vi "Math Algos 2.vi"(9 "Measurements 2":T1, 11 "W (from Top View Algo)":dbl[](array[numeric]) format="%#_13g") -> (3 "H corrected":dbl[](array[numeric]))   [LabVIEW 2019, in "Algorithm.lvclass"]
uses:
  FrameworkOverrides/Algorithm.lvclass
  Controls/Measurements JSON Read.ctl
panel:
  out "NumericAray":i32[][](array[numeric])
  out "MeasurementIndices":i32[][](array[numeric])
  out "Array":string[](array[string])
  out "Alpha":dbl[](array[numeric])
  out "Thickness":dbl[](array[numeric])
  out "CurlGap":dbl[](array[numeric])
  out "Radius":dbl[](array[numeric])
  out "CamID":i32[](array[numeric])=[0, 0, 0, 1, 2, 1, 2, 1, 2, 1, 2, 0, 1, 2, 1, 2]
  out "Htrig":dbl[](array[numeric])
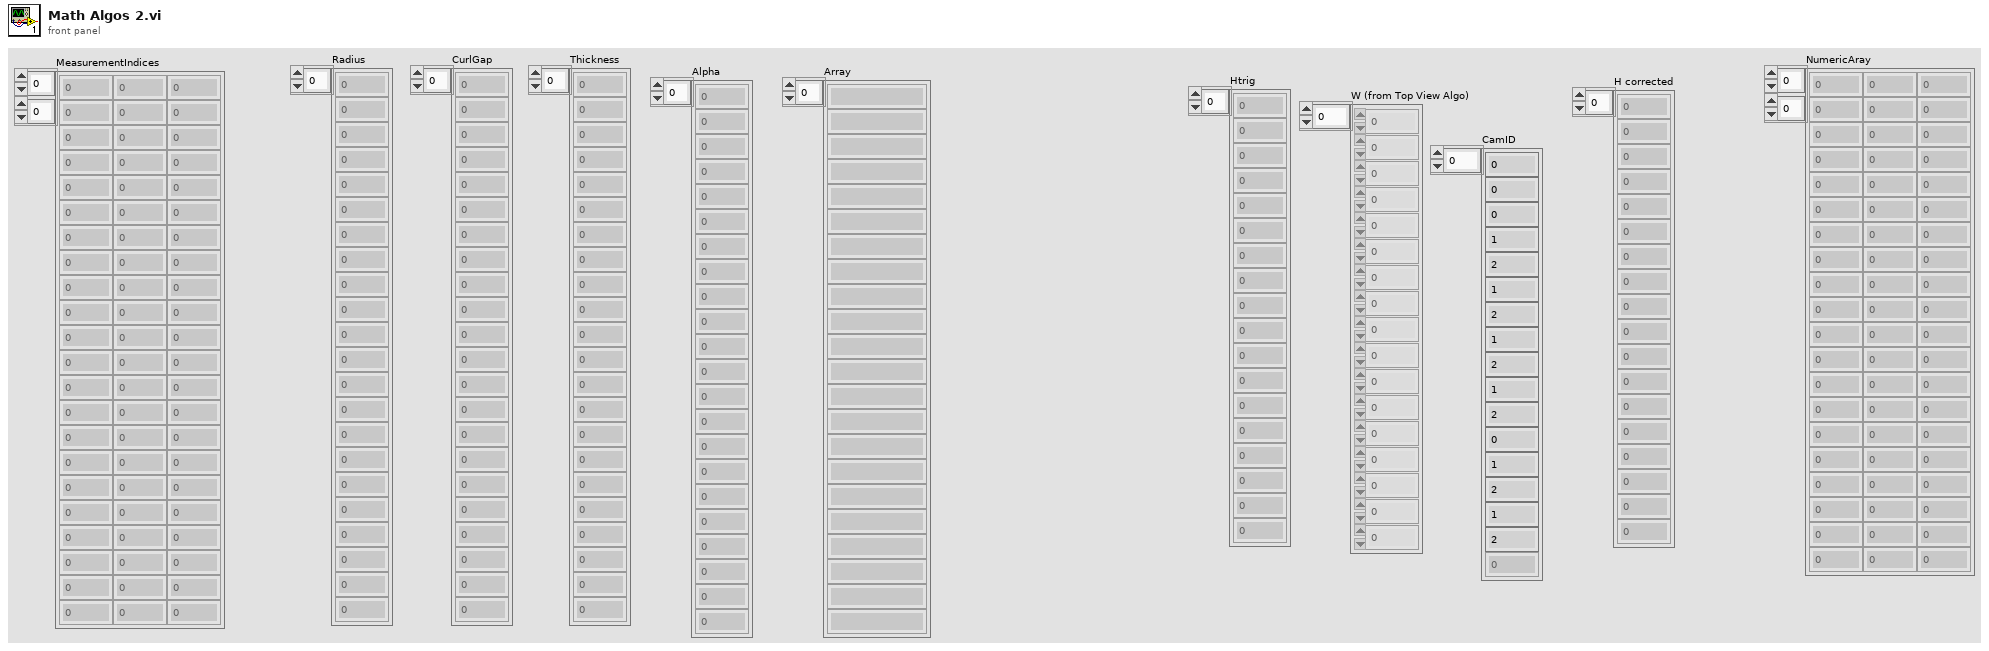
[diagram p1: front panel]
types:
  T1 = typedef "Algorithm.lvclass/Measurements JSON Read.ctl" = cluster{"RackID":i32, "ImageID":i32, "CameraID":i32, "MeasurementId":i32, "Name":string, "AlgoName":string, "Type":string, "MeasurementEnable":bool, "AlgorithmSequence":cluster{"RefernceEdge":cluster{"Enable":bool, "Method":string, "RefROI":cluster{"Left":i32, "Top":i32, "Right":i32, "Bottom":i32, "Rotation":dbl}, "EdgeOptions":cluster{"EdgePoarity":i32, "KernelSize":i32, "Width":i32, "MinimumEdgeStrength":i32, "InterpolationType":i32, "DataProcessingMethod":i32}, "LineOptions":cluster{"NumberofLines":i32, "Type":i32, "MinScore":i32, "MaxScore":i32, "Orientation":i32, "AngleRange":i32, "AngleTolerance":i32, "StepSize":i32, "MinSNR":i32, "MinPoints":i32, "HoughIterations":i32}, "SearchDirection":i32}, "Measurement":cluster{"ROI1":cluster{"Enable":bool, "ROI":cluster{"Left":i32, "Top":i32, "Right":i32, "Bottom":i32, "Rotation":dbl}, "EdgeOptions":cluster{"EdgePoarity":i32, "KernelSize":i32, "Width":i32, "MinimumEdgeStrength":i32, "InterpolationType":i32, "DataProcessingMethod":i32}, "LineOptions":cluster{"NumberofLines":i32, "Type":i32, "MinScore":i32, "MaxScore":i32, "Orientation":i32, "AngleRange":i32, "AngleTolerance":i32, "StepSize":i32, "MinSNR":i32, "MinPoints":i32, "HoughIterations":i32}, "Process":i32, "StepSize":i32, "SearchDirection":i32, "CircleEdgeOptions":cluster{"SearchDirection":i32, "EdgeOptions":cluster{"EdgePoarity":i32, "KernelSize":i32, "Width":i32, "MinimumEdgeStrength":i32, "InterpolationType":i32, "DataProcessingMethod":i32}}, "CircleFitOptions":cluster{"Process":i32, "StepSize":i32, "MAxPixelRadius":dbl}, "CircleSearchDirection":i32, "CurveParameters":cluster{"ExtractionMode":i32, "EdgeThreshold":i32, "EdgeFilterSize":i32, "MinLength":i32, "RowSearchStepSize":i32, "ColSearchStepSize":i32, "MaxEndpointGap":i32, "Closed":bool, "Subpixel":bool}, "MinimumMatchScore":i32, "CircleDescriptor":cluster{"MinRadius":i32, "MaxRadius":i32}, "EllipseDescriptor":cluster{"MinMajorRadius":i32, "MaxMajorRadius":i32, "MinMinorRadius":i32, "MaxMinorRadius":i32}}, "ROI2":cluster{"Enable":bool, "ROI":cluster{"Left":i32, "Top":i32, "Right":i32, "Bottom":i32, "Rotation":dbl}, "EdgeOptions":cluster{"EdgePoarity":i32, "KernelSize":i32, "Width":i32, "MinimumEdgeStrength":i32, "InterpolationType":i32, "DataProcessingMethod":i32}, "LineOptions":cluster{"NumberofLines":i32, "Type":i32, "MinScore":i32, "MaxScore":i32, "Orientation":i32, "AngleRange":i32, "AngleTolerance":i32, "StepSize":i32, "MinSNR":i32, "MinPoints":i32, "HoughIterations":i32}, "Process":i32, "StepSize":i32, "SearchDirection":i32, "CircleEdgeOptions":cluster{"SearchDirection":i32, "EdgeOptions":cluster{"EdgePoarity":i32, "KernelSize":i32, "Width":i32, "MinimumEdgeStrength":i32, "InterpolationType":i32, "DataProcessingMethod":i32}}, "CircleFitOptions":cluster{"Process":i32, "StepSize":i32, "MAxPixelRadius":dbl}, "CircleSearchDirection":i32, "CurveParameters":cluster{"ExtractionMode":i32, "EdgeThreshold":i32, "EdgeFilterSize":i32, "MinLength":i32, "RowSearchStepSize":i32, "ColSearchStepSize":i32, "MaxEndpointGap":i32, "Closed":bool, "Subpixel":bool}, "MinimumMatchScore":i32, "CircleDescriptor":cluster{"MinRadius":i32, "MaxRadius":i32}, "EllipseDescriptor":cluster{"MinMajorRadius":i32, "MaxMajorRadius":i32, "MinMinorRadius":i32, "MaxMinorRadius":i32}}}}, "MathExpression":cluster{"Algorithm":string, "MathExpression":string, "ResultVariable":string}, "MathCorrectionParameters":cluster{"Radius":dbl, "CurlGap":dbl, "Thickness":dbl, "MeasurementIndices":i32[], "MathAlgoName":string, "MathAlgoFormula":string, "CorrectionForAngle":i32[], "NumericAray":i32[], "StringArray":string[]}, "ResultVariableCluster":cluster{"RVName":string, "RVSequence":string, "RVIndex":i32, "RVID":i32, "RVValue":dbl}, "CalibrationCoefficients":cluster{"A1":dbl, "A2":dbl, "A3":dbl}, "UserCalibCoefficients":cluster{"UserCorrectionLinearityCoeff":dbl, "UserCorrectionBiasCoeff":dbl}, "SpecValues":cluster{"LCL":dbl, "UCL":dbl, "LSL":dbl, "USL":dbl, "NominalValue":dbl}, "OverlayOptions":cluster{"OverlayEnable":bool, "OverlayText":string, "OverlayCoords":i32[], "OverlayAngle":i32, "OverlayTextSize":i32, "OverlayTextColor":string, "OverlayROI":bool, "OverlayRakeLine":bool, "OverlayPoints":bool}, "DatalogEnable":bool, "DisplayIcon":string}[]
  T2 = cluster{"Radius":dbl, "CurlGap":dbl, "Thickness":dbl, "MeasurementIndices":i32[], "MathAlgoName":string, "MathAlgoFormula":string, "CorrectionForAngle":i32[], "NumericAray":i32[], "StringArray":string[]}
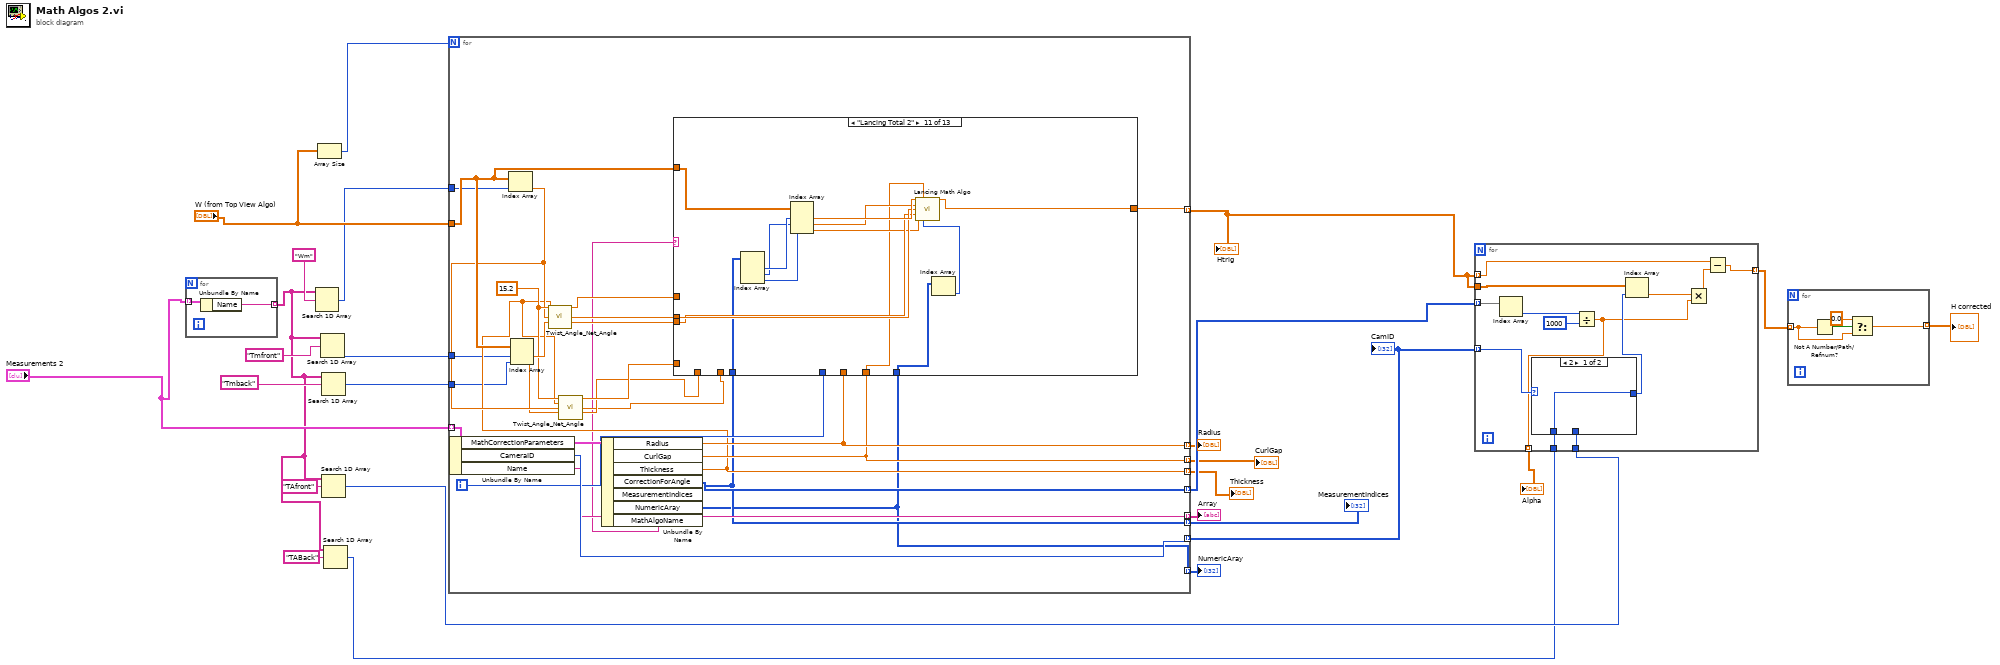
[diagram p0: block diagram]
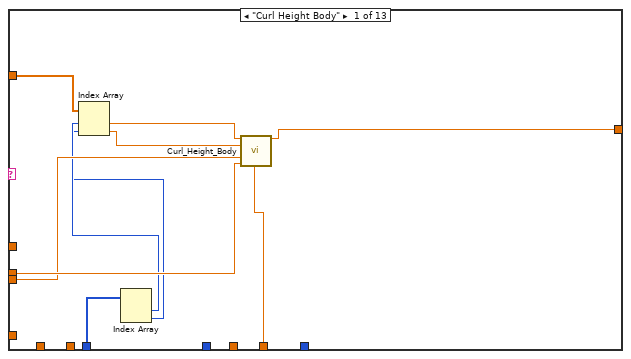
[diagram p3: hidden frame]
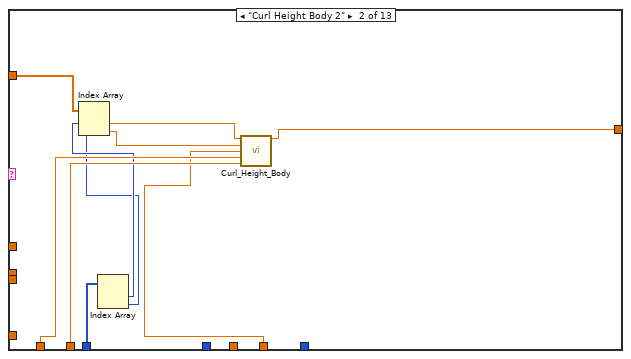
[diagram p4: hidden frame]
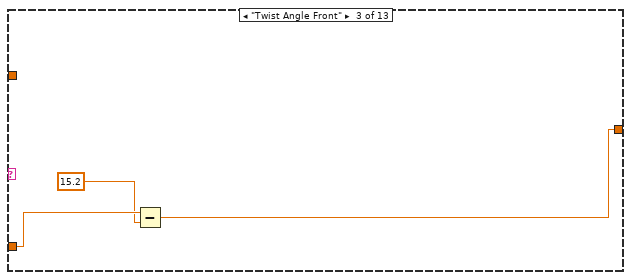
[diagram p5: hidden frame]
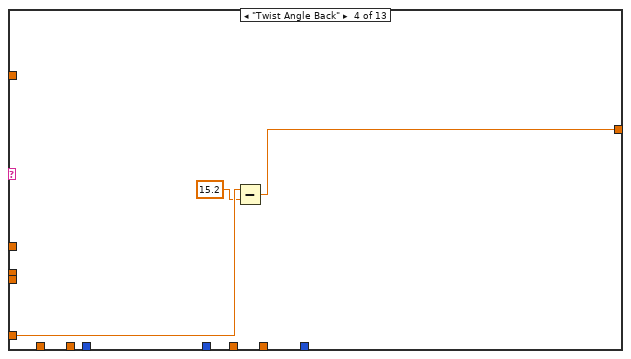
[diagram p6: hidden frame]
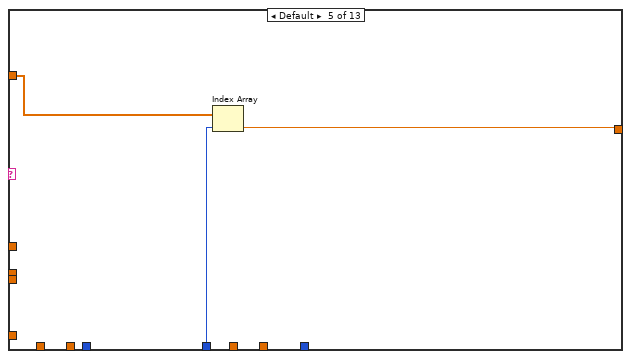
[diagram p7: hidden frame]
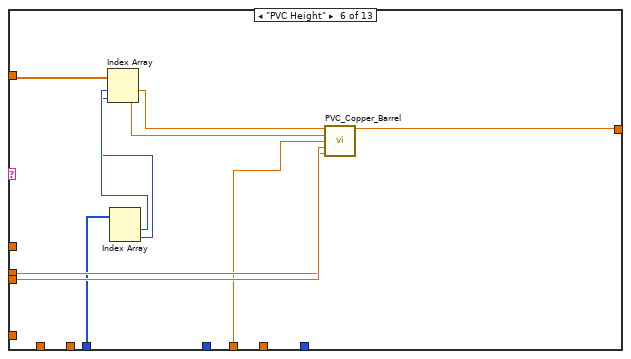
[diagram p8: hidden frame]
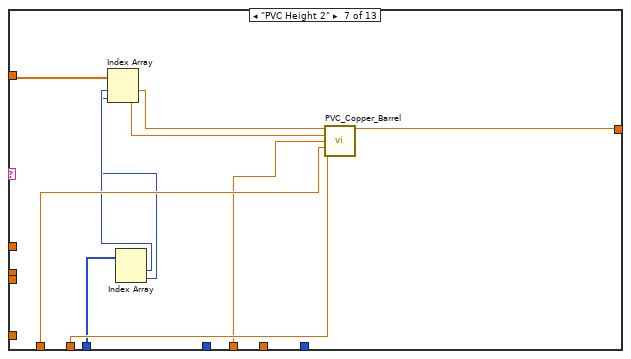
[diagram p9: hidden frame]
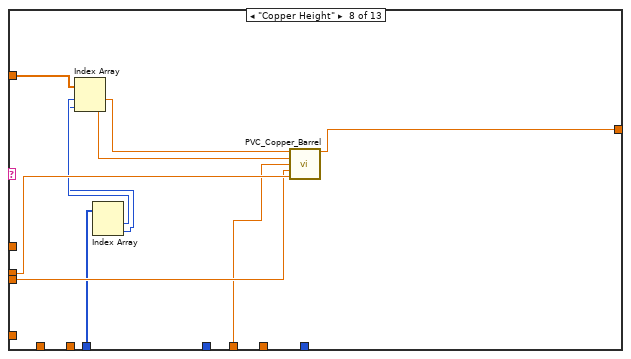
[diagram p10: hidden frame]
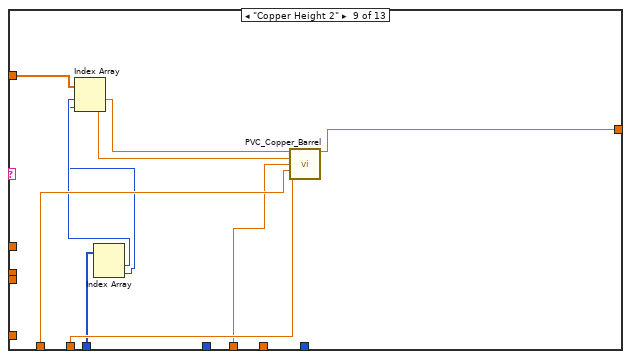
[diagram p11: hidden frame]
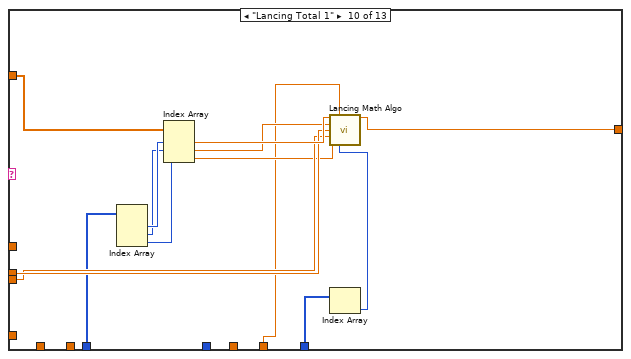
[diagram p12: hidden frame]
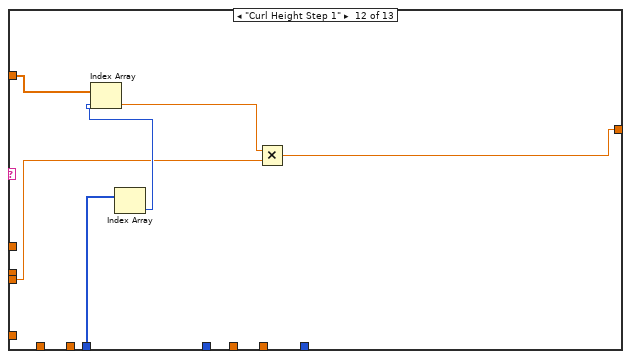
[diagram p13: hidden frame]
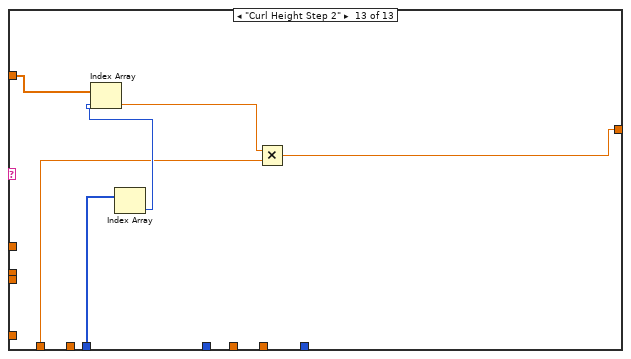
[diagram p14: hidden frame]
diagram:
  n1 = for {
    tunnel: "Measurements 2" -> [w28] mode=indexing
    tunnel: [w27] -> w5 mode=indexing
    n2 = Unbundle By Name(w28) -> ("Name"=w27:string)
  }
  n3 = Search 1D Array(1D array=w5, element="Wm") -> (index of element=w11:i32)  [unwired: 1 in]
  n4 = Array Size(array="W (from Top View Algo)") -> (size(s)=w26:i32)
  n5 = Search 1D Array(1D array=w5, element="Tmfront") -> (index of element=w9:i32)  [unwired: 1 in]
  n6 = Search 1D Array(1D array=w5, element="Tmback") -> (index of element=w7:i32)  [unwired: 1 in]
  n7 = Search 1D Array(1D array=w5, element="TAfront") -> (index of element=w3:i32)  [unwired: 1 in]
  n8 = Search 1D Array(1D array=w5, element="TABack") -> (index of element=w2:i32)  [unwired: 1 in]
  n9 = for {
    N: w26 -> [_]
    tunnel: "W (from Top View Algo)" -> [w55]
    tunnel: [w52] -> w24 mode=indexing
    tunnel: "Measurements 2" -> [w43] mode=indexing
    tunnel: [w41] -> w21 mode=indexing
    tunnel: [w40] -> w20 mode=indexing
    tunnel: [w38] -> w19 mode=indexing
    tunnel: [w37] -> w18 mode=indexing
    tunnel: [w36] -> w17 mode=indexing
    tunnel: [w35] -> w15 mode=indexing
    tunnel: [w34] -> w14 mode=indexing
    tunnel: w11 -> [w33]
    tunnel: w9 -> [w32]
    tunnel: w7 -> [w31]
    tunnel: [w30] -> w1 mode=indexing
    i -> [w39]
    w46 = 15.2 ("Theta_c")
    n10 = Unbundle By Name(w43) -> ("MathCorrectionParameters"=w42:T2, "CameraID"=w41:i32, "Name"=w35:string)
    n11 = Index Array(array=w55, index=w33) -> (element=w45:dbl)
    n12 = Index Array(array=w55, index #1=w32, index #2=w31) -> (element #1=w50:dbl, element #2=w44:dbl)
    n13 = Unbundle By Name(w42) -> ("Radius"=w38:dbl, "CurlGap"=w37:dbl, "Thickness"=w36:dbl, "CorrectionForAngle"=w40:i32[], "MeasurementIndices"=w34:i32[], "NumericAray"=w30:i32[], "MathAlgoName"=w29:string)
    n14 = call "Twist_Angle_Net_Angle.vi"("Theta_c"=w46, "Neck Thickness"=w36, "Wm"=w45, "Tm"=w50) -> ("Net"=w51:dbl, "Sine_Net"=w54:dbl, "Cosine_Net"=w53:dbl)  [unwired: 8 in, 1 out]
    n15 = call "Twist_Angle_Net_Angle.vi"("Theta_c"=w46, "Neck Thickness"=w36, "Wm"=w45, "Tm"=w44) -> ("Net"=w49:dbl, "Sine_Net"=w47:dbl, "Cosine_Net"=w48:dbl)  [unwired: 8 in, 1 out]
    n16 = case shown="\"Lancing Total 2\"" w29 {
      tunnel: w55 -> [w65 w75 _ _ w83 w93 w103 w113 w123 w138 w152 w158 w164]
      tunnel: w54 -> [w62 _ _ _ _ w89 _ w110 _ w135 w149 _ _]
      tunnel: w53 -> [w61 _ _ _ _ w90 _ w109 _ w134 w148 w153 _]
      tunnel: [w60 w72 w78 w81 w82 w94 w104 w114 w124 w132 w146 w154 w160] -> w52
      tunnel: w39 -> [_ _ _ _ w84 _ _ _ _ _ _ _ _]
      tunnel: w51 -> [_ _ w77 _ _ _ _ _ _ _ _ _ _]
      tunnel: w49 -> [_ _ _ w80 _ _ _ _ _ _ _ _ _]
      tunnel: w48 -> [_ w70 _ _ _ _ w100 _ w120 _ _ _ w159]
      tunnel: w47 -> [_ w71 _ _ _ _ w99 _ w119 _ _ _ _]
      tunnel: w38 -> [_ _ _ _ _ w88 w98 w108 w118 _ _ _ _]
      tunnel: w37 -> [w59 w69 _ _ _ _ _ _ _ w131 w145 _ _]
      tunnel: w34 -> [w58 w68 _ _ _ w87 w97 w107 w117 w130 w144 w157 w163]
      tunnel: w30 -> [_ _ _ _ _ _ _ _ _ w126 w140 _ _]
      frame "Curl Height Body" {
        n17 = Index Array(array=w58) -> (element #1=w57:i32, element #2=w56:i32)  [unwired: 2 in]
        n18 = Index Array(array=w65, index #1=w57, index #2=w56) -> (element #1=w64:dbl, element #2=w63:dbl)
        n19 = call "Curl_Height_Body.vi"("Wm"=w64, "Hm"=w63, "Curl Gap"=w59, "cos_net"=w61, "sin_net"=w62) -> ("H"=w60:dbl)  [unwired: 10 in]
      }
      frame "Curl Height Body 2" {
        n20 = Index Array(array=w68) -> (element #1=w67:i32, element #2=w66:i32)  [unwired: 2 in]
        n21 = Index Array(array=w75, index #1=w67, index #2=w66) -> (element #1=w74:dbl, element #2=w73:dbl)
        n22 = call "Curl_Height_Body.vi"("Wm"=w74, "Hm"=w73, "Curl Gap"=w69, "cos_net"=w70, "sin_net"=w71) -> ("H"=w72:dbl)  [unwired: 10 in]
      }
      frame "Twist Angle Front" {
        n23 = Subtract(x=w77, y=15.2) -> (x-y=w78:dbl)
      }
      frame "Twist Angle Back" {
        n24 = Subtract(x=w80, y=15.2 ("x")) -> (x-y=w81:dbl)
      }
      frame Default {
        n25 = Index Array(array=w83, index=w84) -> (element=w82:dbl)
      }
      frame "PVC Height" {
        n26 = Index Array(array=w87) -> (element #1=w86:i32, element #2=w85:i32)  [unwired: 2 in]
        n27 = Index Array(array=w93, index #1=w86, index #2=w85) -> (element #1=w92:dbl, element #2=w91:dbl)
        n28 = call "PVC_Copper_Barrel.vi"("Wm"=w92, "Hm"=w91, "R"=w88, "Cos_net"=w90, "Sin_net"=w89) -> ("height"=w94:dbl)  [unwired: 10 in]
      }
      frame "PVC Height 2" {
        n29 = Index Array(array=w97) -> (element #1=w96:i32, element #2=w95:i32)  [unwired: 2 in]
        n30 = Index Array(array=w103, index #1=w96, index #2=w95) -> (element #1=w102:dbl, element #2=w101:dbl)
        n31 = call "PVC_Copper_Barrel.vi"("Wm"=w102, "Hm"=w101, "R"=w98, "Cos_net"=w100, "Sin_net"=w99) -> ("height"=w104:dbl)  [unwired: 10 in]
      }
      frame "Copper Height" {
        n32 = Index Array(array=w107) -> (element #1=w106:i32, element #2=w105:i32)  [unwired: 2 in]
        n33 = Index Array(array=w113, index #1=w106, index #2=w105) -> (element #1=w112:dbl, element #2=w111:dbl)
        n34 = call "PVC_Copper_Barrel.vi"("Wm"=w112, "Hm"=w111, "R"=w108, "Cos_net"=w109, "Sin_net"=w110) -> ("height"=w114:dbl)  [unwired: 10 in]
      }
      frame "Copper Height 2" {
        n35 = Index Array(array=w117) -> (element #1=w116:i32, element #2=w115:i32)  [unwired: 2 in]
        n36 = Index Array(array=w123, index #1=w116, index #2=w115) -> (element #1=w122:dbl, element #2=w121:dbl)
        n37 = call "PVC_Copper_Barrel.vi"("Wm"=w122, "Hm"=w121, "R"=w118, "Cos_net"=w120, "Sin_net"=w119) -> ("height"=w124:dbl)  [unwired: 10 in]
      }
      frame "Lancing Total 1" {
        n38 = Index Array(array=w130) -> (element #1=w129:i32, element #2=w128:i32, element #3=w127:i32)  [unwired: 3 in]
        n39 = Index Array(array=w138, index #1=w129, index #2=w128, index #3=w127) -> (element #1=w137:dbl, element #2=w136:dbl, element #3=w133:dbl)
        n40 = Index Array(array=w126) -> (element=w125:i32)  [unwired: 1 in]
        n41 = call "Lancing Math Algo.vi"("Wm"=w137, "Curl Gap"=w131, "Hm"=w136, "sin_net"=w135, "cos_net"=w134, "Hm'"=w133, "Lock Width"=w125) -> ("Lancing"=w132:dbl)  [unwired: 8 in]
      }
      frame "Lancing Total 2" {
        n42 = Index Array(array=w144) -> (element #1=w143:i32, element #2=w142:i32, element #3=w141:i32)  [unwired: 3 in]
        n43 = Index Array(array=w152, index #1=w143, index #2=w142, index #3=w141) -> (element #1=w151:dbl, element #2=w150:dbl, element #3=w147:dbl)
        n44 = Index Array(array=w140) -> (element=w139:i32)  [unwired: 1 in]
        n45 = call "Lancing Math Algo.vi"("Wm"=w151, "Curl Gap"=w145, "Hm"=w150, "sin_net"=w149, "cos_net"=w148, "Hm'"=w147, "Lock Width"=w139) -> ("Lancing"=w146:dbl)  [unwired: 8 in]
      }
      frame "Curl Height Step 1" {
        n46 = Index Array(array=w157) -> (element=w156:i32)  [unwired: 1 in]
        n47 = Index Array(array=w158, index=w156) -> (element=w155:dbl)
        n48 = Multiply(x=w155, y=w153) -> (x*y=w154:dbl)
      }
      frame "Curl Height Step 2" {
        n49 = Index Array(array=w163) -> (element=w162:i32)  [unwired: 1 in]
        n50 = Index Array(array=w164, index=w162) -> (element=w161:dbl)
        n51 = Multiply(x=w161, y=w159) -> (x*y=w160:dbl)
      }
    }
  }
  "Htrig" <- w24
  "CamID" <- w21
  "Radius" <- w19
  "CurlGap" <- w18
  "Thickness" <- w17
  "Array" <- w15
  "MeasurementIndices" <- w14
  "NumericAray" <- w1
  n52 = for {
    tunnel: w21 -> [w177] mode=indexing
    tunnel: w20 -> [w170] mode=indexing
    tunnel: w24 -> [w174] mode=indexing
    tunnel: w24 -> [w176]
    tunnel: [w171] -> w23 mode=indexing
    tunnel: [w167] -> w16 mode=indexing
    tunnel: w3 -> [w166]
    tunnel: w2 -> [w165]
    n53 = Index Array(array=w170) -> (element=w168:i32)  [unwired: 1 in]
    n54 = case shown="2" w177 {
      tunnel: [w178 w179] -> w175
      tunnel: w166 -> [_ w179]
      tunnel: w165 -> [w178 _]
      frame 2 {
      }
      frame 1, Default {
      }
    }
    n55 = Divide(x=w168, y=1000) -> (x/y=w167:dbl)
    n56 = Index Array(array=w176, index=w175) -> (element=w173:dbl)
    n57 = Multiply(x=w173, y=w167) -> (x*y=w172:dbl)
    n58 = Subtract(x=w174, y=w172) -> (x-y=w171:dbl)
  }
  "Alpha" <- w16
  n59 = for {
    tunnel: w23 -> [w182] mode=indexing
    tunnel: [w180] -> w22 mode=indexing
    n60 = Not A Number/Path/Refnum?(number/path/refnum=w182) -> (NaN/Path/Refnum?=w183:bool)
    n61 = Select(t=0.0, s=w183, f=w182) -> (s? t:f=w180:dbl)
  }
  "H corrected" <- w22
